vi "Swerve Go To.vi"(0 "Max Speed":dbl, 1 "Target X":dbl, 2 "Target Y":dbl, 3 "Target Angle":dbl) -> (6 "Done":bool)   [LabVIEW 2016]
uses:
  <vilib>/addons/control/pid/NI_PID_pid.lvlib
  <vilib>/addons/control/pid/pid.llb/PID (DBL).vi
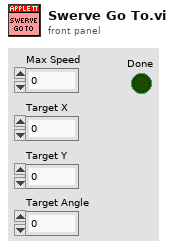
[diagram p1: front panel]
types:
  T1 = enum16{"Prepare to Rotate", "Rotate", "Prepare to Move", "Move"}
  T2 = cluster{"proportional gain (Kc)":dbl, "integral time (Ti, min)":dbl, "derivative time (Td, min)":dbl}
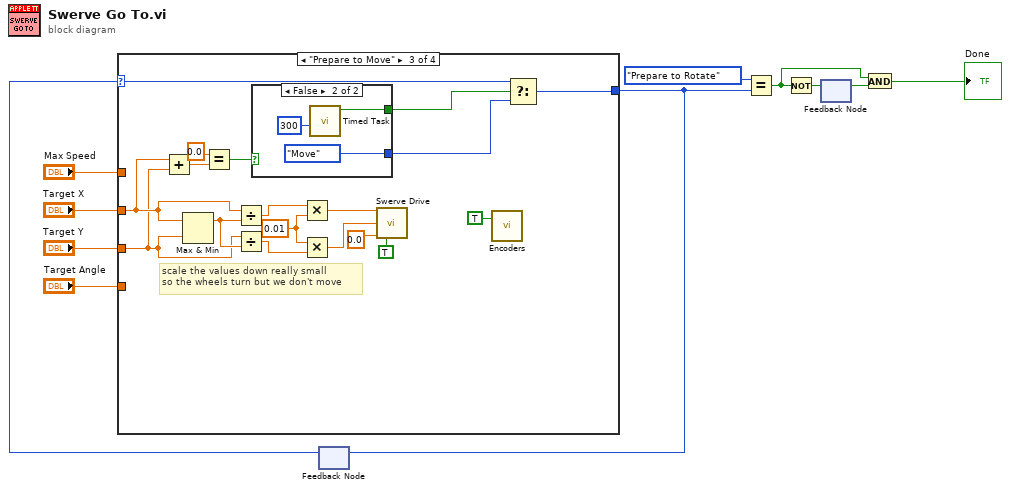
[diagram p0: block diagram]
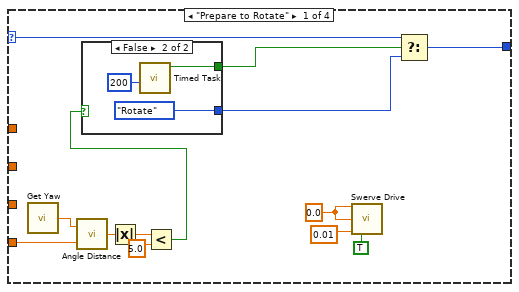
[diagram p2: hidden frame]
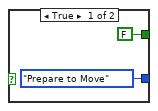
[diagram p3: hidden frame]
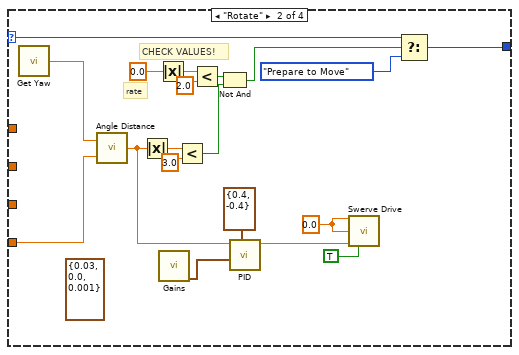
[diagram p4: hidden frame]
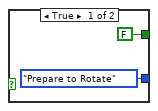
[diagram p5: hidden frame]
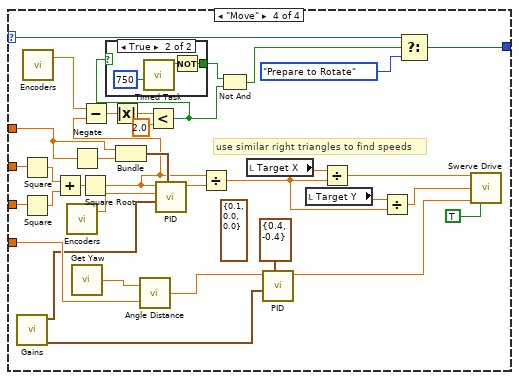
[diagram p6: hidden frame]
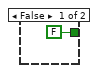
[diagram p7: hidden frame]
diagram:
  n1 = feedback #1() -> (w6:T1)  [unwired: 1 in]
  n2 = case shown="\"Prepare to Move\"" w6 {
    selector: w6 -> [w23 w47 w65 w104]
    tunnel: [w24 w48 w66 w105] -> w1
    tunnel: "Target Angle" -> [w20 w35 _ w87]
    tunnel: "Target X" -> [_ _ w57 w102]
    tunnel: "Target Y" -> [_ _ w56 w101]
    tunnel: "Max Speed" -> [_ _ _ w95]
    frame "Prepare to Rotate" {
      w22 = 0.0
      n3 = call "Get Yaw.vi"() -> ("Angle"=w12:dbl)  [unwired: 1 in]
      n4 = call "Angle Distance.vi"("target angle"=w20, "current angle"=w12) -> ("distance"=w19:dbl)
      n5 = Absolute Value(x=w19) -> (abs(x)=w18:dbl)
      n6 = Less?(x=w18, y=5.0) -> (x < y?=w16:bool)
      n7 = case shown="False" w16 {
        tunnel: [FALSE w28] -> w14
        tunnel: [T1."Prepare to Move" T1."Rotate"] -> w15
        frame True {
        }
        frame False, Default {
          n8 = call "Timed Task.vi"("Time (ms)"=u32 200) -> ("Running"=w28:bool)  [unwired: 10 in]
        }
      }
      n9 = call "Swerve Drive.vi"("X"=w22, "Y"=w22, "Z"=0.01, "Auto Controls"=TRUE) -> ()  [unwired: 12 in]
      n10 = Select(t=w23, s=w14, f=w15) -> (s? t:f=w24:T1)
    }
    frame "Rotate" {
      (unwired) T2 {"proportional gain (Kc)"=0.03, "integral time (Ti, min)"=0.0, "derivative time (Td, min)"=0.001} ("PID gains")
      w45 = 0.0
      # "rate"
      # "CHECK VALUES!"
      n11 = call "Get Yaw.vi"() -> ("Angle"=w32:dbl)  [unwired: 1 in]
      n12 = call "Angle Distance.vi"("target angle"=w35, "current angle"=w32) -> ("distance"=w34:dbl)
      n13 = Absolute Value(x=w34) -> (abs(x)=w40:dbl)
      n14 = Absolute Value(x=0.0) -> (abs(x)=w43:dbl)
      n15 = call "Gains.vi"() -> ("Rot"=w30:T2)  [unwired: 10 in, 1 out]
      n16 = Less?(x=w40, y=3.0) -> (x < y?=w37:bool)
      n17 = Less?(x=w43, y=2.0) -> (x < y?=w39:bool)
      n18 = Not And(1:w37, 2:w39) -> (0:w38:bool)
      n19 = call-poly <vilib>:"PID.vi"("output range"=cluster{"output high":dbl, "output low":dbl} {"output high"=0.4, "output low"=-0.4}, "PID gains"=w30, "setpoint"=w34) -> ("output"=w36:dbl)  [unwired: 7 in, 1 out]
      n20 = call "Swerve Drive.vi"("X"=w45, "Y"=w45, "Z"=w36, "Auto Controls"=TRUE) -> ()  [unwired: 12 in]
      n21 = Select(t=w47, s=w38, f=T1."Prepare to Move") -> (s? t:f=w48:T1)
    }
    frame "Prepare to Move" {
      w63 = 0.01 ("y")
      # "scale the values down really small\nso the wheels turn but we don't move"
      n22 = Add(x=w57, y=w56) -> (x+y=w55:dbl)
      n23 = Max & Min(x=w57, y=w56) -> (max(x,y)=w64:dbl)  [unwired: 1 out]
      n24 = Equal?(x=0.0, y=w55) -> (x = y?=w53:bool)
      n25 = Divide(x=w57, y=w64) -> (x/y=w61:dbl)
      n26 = Divide(x=w56, y=w64) -> (x/y=w62:dbl)
      n27 = case shown="False" w53 {
        tunnel: [FALSE w70] -> w51
        tunnel: [T1."Prepare to Rotate" T1."Move"] -> w52
        frame True {
        }
        frame False, Default {
          n28 = call "Timed Task.vi"("Time (ms)"=u32 300) -> ("Running"=w70:bool)  [unwired: 10 in]
        }
      }
      n29 = Multiply(x=w61, y=w63) -> (x*y=w60:dbl)
      n30 = Multiply(x=w63, y=w62) -> (x*y=w59:dbl)
      n31 = call "Swerve Drive.vi"("X"=w60, "Y"=w59, "Z"=0.0, "Auto Controls"=TRUE) -> ()  [unwired: 12 in]
      n32 = call "Encoders.vi"("Reset All"=TRUE) -> ()  [unwired: 1 in, 2 out]
      n33 = Select(t=w65, s=w51, f=w52) -> (s? t:f=w66:T1)
    }
    frame "Move" {
      (unwired) T2 {"proportional gain (Kc)"=0.1, "integral time (Ti, min)"=0.0, "derivative time (Td, min)"=0.0} ("PID gains")
      # "use similar right triangles to find speeds"
      n34 = call "Gains.vi"() -> ("Rot"=w73:T2, "Drive"=w72:T2)  [unwired: 10 in]
      n35 = Square(x=w102) -> (x^2=w100:dbl)
      n36 = Square(x=w101) -> (x^2=w99:dbl)
      n37 = call "Encoders.vi"() -> ("Avg Absolute Distance"=w84:dbl)  [unwired: 2 in, 1 out]
      n38 = Add(x=w100, y=w99) -> (x+y=w98:dbl)
      n39 = call "Encoders.vi"() -> ("Avg Absolute Distance"=w88:dbl)  [unwired: 2 in, 1 out]
      n40 = Negate(x=w95) -> (-x=w96:dbl)
      n41 = call "Get Yaw.vi"() -> ("Angle"=w83:dbl)  [unwired: 1 in]
      n42 = Square Root(x=w98) -> (sqrt(x)=w81:dbl)
      n43 = Subtract(x=w84, y=w81) -> (x-y=w92:dbl)
      n44 = Absolute Value(x=w92) -> (abs(x)=w93:dbl)
      n45 = Bundle("Max Speed"=w95, w96) -> (w97:cluster{"Max Speed":dbl, dbl})  [unwired: 1 in]
      n46 = call "Angle Distance.vi"("target angle"=w87, "current angle"=w83) -> ("distance"=w86:dbl)
      n47 = Less?(x=w93, y=2.0) -> (x < y?=w74:bool)
      n48 = case shown="True" w74 {
        tunnel: [FALSE w108] -> w75
        frame False {
        }
        frame True {
          n49 = call "Timed Task.vi"("Time (ms)"=750) -> ("Running"=w109:bool)  [unwired: 10 in]
          n50 = Not(x=w109) -> (.not. x?=w108:bool)
        }
      }
      n51 = call-poly <vilib>:"PID.vi"("output range"=w97, "PID gains"=w72, "process variable"=w88, "setpoint"=w81) -> ("output"=w82:dbl)  [unwired: 6 in, 1 out]
      n52 = Divide(x=w81, y=w82) -> (x/y=w79:dbl)
      n53 = Not And(1:w74, 2:w75) -> (0:w91:bool)
      n54 = local read "Target X"() -> (w80:dbl)
      n55 = call-poly <vilib>:"PID.vi"("output range"=cluster{"output high":dbl, "output low":dbl} {"output high"=0.4, "output low"=-0.4}, "PID gains"=w73, "setpoint"=w86) -> ("output"=w89:dbl)  [unwired: 7 in, 1 out]
      n56 = local read "Target Y"() -> (w78:dbl)
      n57 = Divide(x=w80, y=w79) -> (x/y=w76:dbl)
      n58 = Divide(x=w78, y=w79) -> (x/y=w77:dbl)
      n59 = Select(t=w104, s=w91, f=T1."Prepare to Rotate") -> (s? t:f=w105:T1)
      n60 = call "Swerve Drive.vi"("X"=w76, "Y"=w77, "Z"=w89, "Auto Controls"=TRUE) -> ()  [unwired: 12 in]
    }
  }
  n61 = feedback-in #1(w1) -> ()
  n62 = Equal?(x=T1."Prepare to Rotate", y=w1) -> (x = y?=w2:bool)
  n63 = Not(x=w2) -> (.not. x?=w4:bool)
  n64 = feedback #2() -> (w3:bool)  [unwired: 1 in]
  n65 = feedback-in #2(w4) -> ()
  n66 = And(x=w2, y=w3) -> (x .and. y?=→"Done":bool)
